vi "Format Attribute.vi"(5 "Attribute Names":string[](array[string]), 6 "Indent":i32, 7 "Attribute Values":variant[](array[variant]), 11 "XML in":refnum<class "XML.lvclass">) -> (3 "XML out":refnum<class "XML.lvclass">, 4 "Attr Strings":string[](array[string]))   [LabVIEW 2020, in "XML.lvlib" / "XML.lvclass"]
uses:
  <vilib>/gpm_packages/@cs/persistence/source/XML/XML.lvclass
  <vilib>/gpm_packages/@cs/persistence/source/XML/XML.lvclass/XML.ctl
  <vilib>/Utility/Data Type/NI_Data Type.lvlib
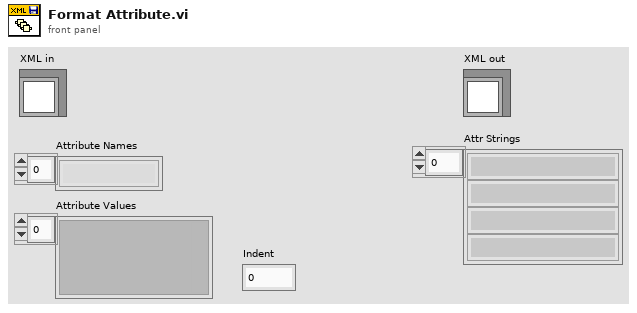
[diagram p1: front panel]
types:
  T1 = typedef "NI_Data Type.lvlib/Data Type.ctl" = enum8{"Invalid Type", "Void", "I8", "I16", "I32", "I64", "U8", "U16", "U32", "U64", "Single Float", "Double Float", "Extended Float", "Single Complex", "Double Complex", "Extended Complex", "Enum U8", "Enum U16", "Enum U32", "Enum U64", "Single Float With Unit", "Double Float With Unit", "Extended Float With Unit", "Single Complex with Unit", "Double Complex with Unit", "Extended Complex with Unit", "Boolean", "String", "Path", "Picture", "Tag", "Array", "Cluster", "Variant", "LV Variant", "Waveform", "Timestamp", "Digital Waveform", "Digital Data", "ExpressData", "Refnum", "External Data", "VI", "Poly VI", "LabVIEW Class Instance", "Fixed Point", "Set Collection", "Map Collection"}
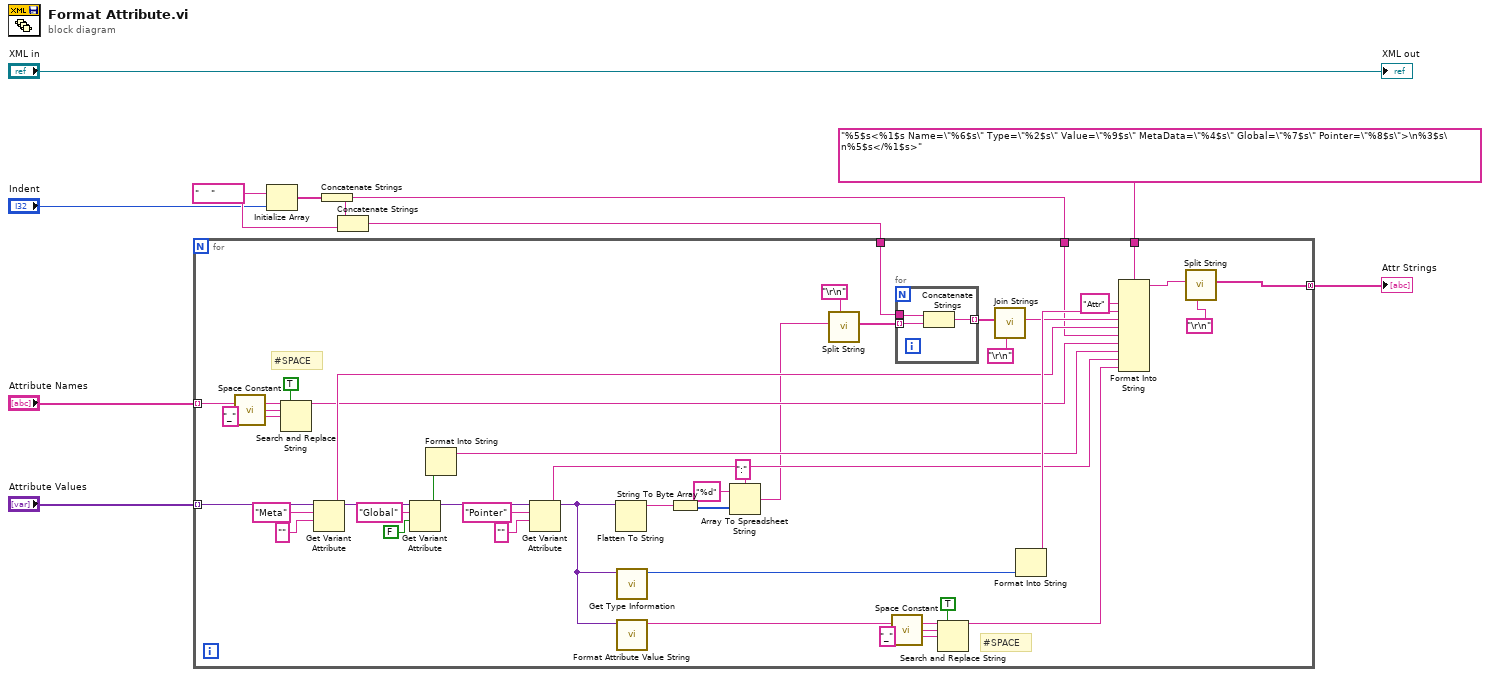
[diagram p0: block diagram]
diagram:
  w9 = "    "
  n1 = Initialize Array(w9, "Indent") -> (w10:string[])
  n2 = Concatenate Strings(w10) -> (w8:string)
  n3 = Concatenate Strings(w8, w9) -> (w6:string)
  n4 = for {
    tunnel: "Attribute Names" -> [w50] mode=indexing
    tunnel: "Attribute Values" -> [w47] mode=indexing
    tunnel: w8 -> [w30]
    tunnel: "%5$s<%1$s Name=\"%6$s\" Type=\"%2$s\" Value=\"%9$s\" MetaData=\"%4$s\" Global=\"%7$s\" Pointer=\"%8$s\">\n%3$s\n%5$s</%1$s>" ("format string") -> [w39]
    tunnel: w6 -> [w35]
    tunnel: [w24] -> w2 mode=concatenating
    # "#SPACE"
    # "#SPACE"
    n5 = call <vilib>:"Space Constant.vi"() -> ("String"=w53:string)
    n6 = Search and Replace String(replace all?=TRUE ("replace all? (F)"), input string=w50, search string=w53, replace string="_") -> (result string=w29:string)  [unwired: 4 in, 3 out]
    n7 = Get Variant Attribute(Variant=w47, name="Meta", default value (empty Variant)="") -> (duplicate Variant=w46:variant, value=w31:string)  [unwired: 1 in, 2 out]
    n8 = Get Variant Attribute(Variant=w46, name="Global", default value (empty Variant)=FALSE) -> (duplicate Variant=w42:variant, value=w28:bool)  [unwired: 1 in, 2 out]
    n9 = Format Into String(w28) -> (resulting string=w27:string)  [unwired: 3 in, 1 out]
    n10 = Get Variant Attribute(Variant=w42, name="Pointer", default value (empty Variant)="") -> (duplicate Variant=w21:variant, value=w26:string)  [unwired: 1 in, 2 out]
    n11 = Flatten To String(anything=w21) -> (data string=w15:string)  [unwired: 3 in, 2 out]
    n12 = call <vilib>:"Get Type Information.vi"("variant"=w21) -> ("type"=w49:T1)  [unwired: 6 in, 4 out]
    n13 = call <vilib>:"Format Attribute Value String.vi"("Data"=w21) -> ("Value as String"=w17:string)  [unwired: 9 in, 1 out]
    n14 = String To Byte Array(string=w15) -> (unsigned byte array=w14:u8[])
    n15 = Array To Spreadsheet String(delimiter (Tab)=":", array=w14, 3:"%d" ("format string")) -> (spreadsheet string=w11:string)
    n16 = call <vilib>:"Split String.vi"("Split Pattern"="\r\n", "Input String"=w11) -> ("Split String"=w36:string[])  [unwired: 9 in]
    n17 = call <vilib>:"Space Constant.vi"() -> ("String"=w20:string)
    n18 = for {
      tunnel: w36 -> [w56] mode=indexing
      tunnel: w35 -> [w55]
      tunnel: [w54] -> w34 mode=indexing
      n19 = Concatenate Strings(w55, w56) -> (w54:string)
    }
    n20 = Search and Replace String(replace all?=TRUE ("replace all? (F)"), input string=w17, search string=w20, replace string="_") -> (result string=w16:string)  [unwired: 4 in, 3 out]
    n21 = call <vilib>:"Join Strings.vi"("Separator (,)"="\r\n", "Strings In"=w34) -> ("String"=w32:string)  [unwired: 9 in]
    n22 = Format Into String(w49) -> (resulting string=w37:string)  [unwired: 3 in, 1 out]
    n23 = Format Into String(format string=w39, "Attr" ("input 1"), w37, w32, w31, w30, w29, w27, w26, w16) -> (resulting string=w25:string)  [unwired: 2 in, 1 out]
    n24 = call <vilib>:"Split String.vi"("Split Pattern"="\r\n", "Input String"=w25) -> ("Split String"=w24:string[])  [unwired: 9 in]
  }
  "Attr Strings" <- w2
  "XML out" <- "XML in"
